vi "Main.vi"() -> ()   [LabVIEW 2017]
panel:
  in  "OSU":bool
  in  "PCU":bool
  in  "MPM":bool
  in  "TSL":bool
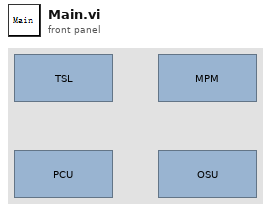
[diagram p1: front panel]
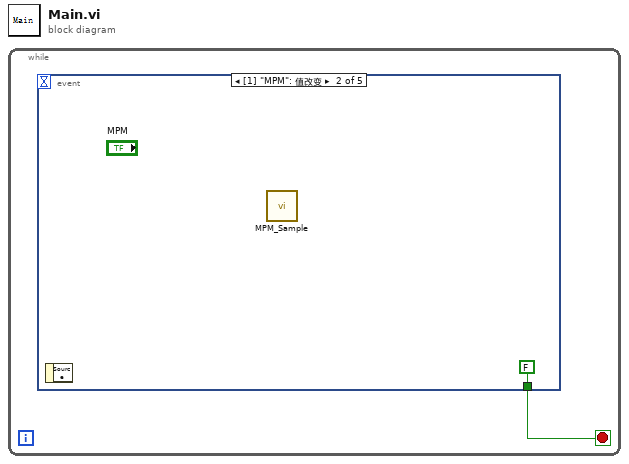
[diagram p0: block diagram]
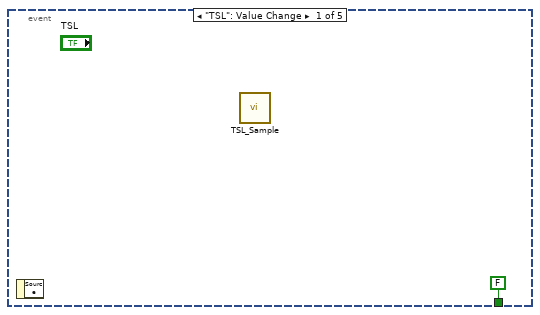
[diagram p2: hidden frame]
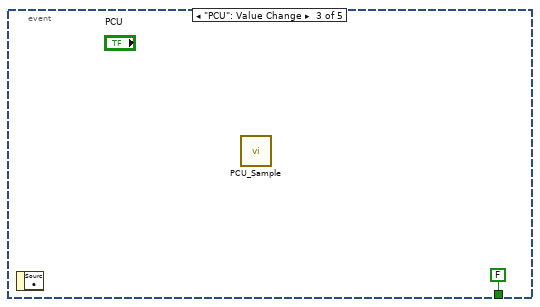
[diagram p3: hidden frame]
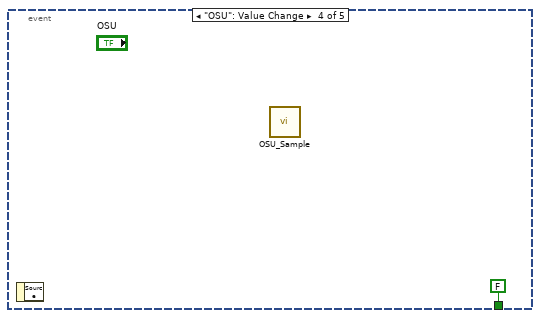
[diagram p4: hidden frame]
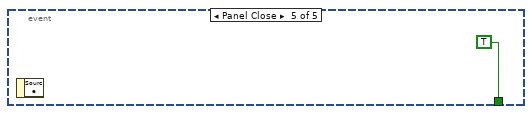
[diagram p5: hidden frame]
diagram:
  n1 = while {
    stop <- w1 stop-if-true
    n2 = event shown="[1] \"MPM\": 值改变" {
      selector: _ -> [_ _ _ _ _]
      dyn-events: _ -> [_ _ _ _ _]
      timeout: _ -> [_ _ _ _ _]
      tunnel: [FALSE FALSE FALSE FALSE TRUE] -> w1
      event "TSL": Value Change {
        n3 = event-data() -> ()  [unwired: 1 in, 1 out]
        n4 = call "TSL_Sample.vi"() -> ()  [unwired: 12 in]
      }
      event "MPM": Value Change {
        n5 = event-data() -> ()  [unwired: 1 in, 1 out]
        n6 = call "MPM_Sample.vi"() -> ()  [unwired: 12 in]
      }
      event "PCU": Value Change {
        n7 = event-data() -> ()  [unwired: 1 in, 1 out]
        n8 = call "PCU_Sample.vi"() -> ()  [unwired: 12 in]
      }
      event "OSU": Value Change {
        n9 = event-data() -> ()  [unwired: 1 in, 1 out]
        n10 = call "OSU_Sample.vi"() -> ()  [unwired: 12 in]
      }
      event Panel Close {
        n11 = event-data() -> ()  [unwired: 1 in, 1 out]
      }
    }
  }
